vi "Error Handler.vi"(8 "error in (no error)":errorcluster, 10 "clear inline error? (F)":bool, 11 "Framework in":refnum<class "Framework.lvclass">) -> (0 "error out":errorcluster, 3 "Framework out":refnum<class "Framework.lvclass">)   [LabVIEW 2017, in "DSF Core.lvlib" / "Framework.lvclass"]
uses:
  Framework.lvclass
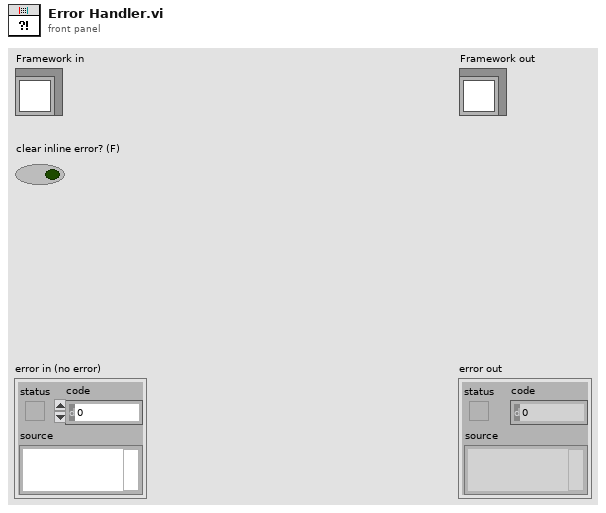
[diagram p1: front panel]
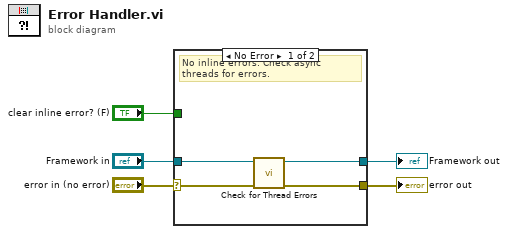
[diagram p0: block diagram]
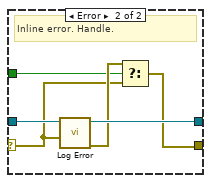
[diagram p2: hidden frame]
diagram:
  n1 = case shown="No Error" "error in (no error)" {
    selector: "error in (no error)" -> [w9 w12]
    tunnel: "Framework in" -> [w8 w15]
    tunnel: [w6 w14] -> w4
    tunnel: [w7 w10] -> w3
    tunnel: "clear inline error? (F)" -> [_ w11]
    frame No Error {
      # "No inline errors. Check async threads for errors."
      n2 = call "Check for Thread Errors.vi"("error in (no error)"=w9, "Framework in"=w8) -> ("error out"=w7:errorcluster, "Framework out"=w6:refnum<class "Framework.lvclass">)  [unwired: 8 in]
    }
    frame Error {
      # "Inline error. Handle."
      n3 = call "Log Error.vi"("error"=w12, "Framework in"=w15) -> ("error out"=w13:errorcluster, "Framework out"=w14:refnum<class "Framework.lvclass">)  [unwired: 8 in]
      n4 = Select(t=w13, s=w11, f=w12) -> (s? t:f=w10:errorcluster)
    }
  }
  "error out" <- w3
  "Framework out" <- w4
